vi "Find project item.vi"(8 "in (no error)":errorcluster, 9 "Item Name":string, 10 "Item Type":string, 11 "Library Refnum In":refnum<vi>) -> (0 "error out":errorcluster, 1 "Path":path, 2 "Project Item":refnum<vi>, 3 "Library Refnum Out":refnum<vi>, 5 "Found ?":bool)   [LabVIEW 2018, in "Palette Generation.lvlib"]
doc: "Find the project item reference for a particular object by name. Also returns the path to the project item."
uses:
  Palette Generation.lvlib
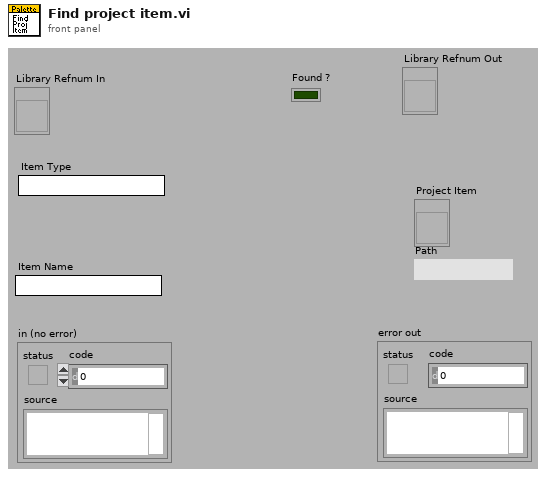
[diagram p1: front panel]
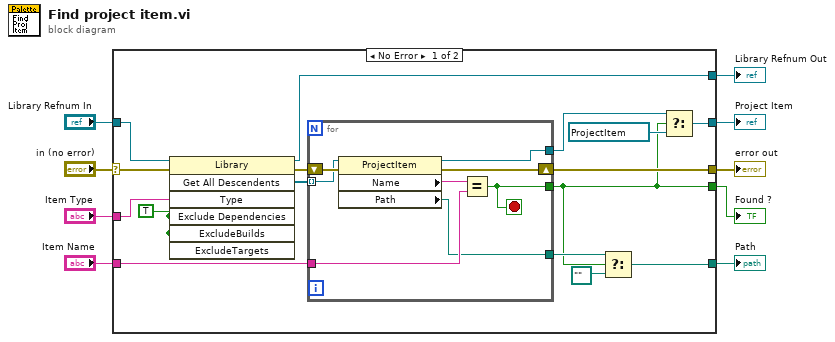
[diagram p0: block diagram]
diagram:
  n1 = case shown="No Error" "in (no error)" {
    selector: "in (no error)" -> [w10 w34]
    tunnel: [w25 w34] -> w9
    tunnel: [w24 _] -> w8
    tunnel: [w23 _] -> w7
    tunnel: "Library Refnum In" -> [w22 _]
    tunnel: "Item Name" -> [w15 _]
    tunnel: "Item Type" -> [w14 _]
    tunnel: [w12 _] -> w2
    tunnel: [w11 _] -> w1
    frame No Error {
      w13 = TRUE ("ExcludeDependencies")
      n2 = invoke class="Library" method="Get All Descendents"(reference=w22, error in=w10, "Type"=w14, "Exclude Dependencies"=w13, "ExcludeBuilds"=w13, "ExcludeTargets"=w13) -> (reference out=w12:refnum<vi>, error out=w21:errorcluster, "All Descendents"=w16:refnum<vi>[])  [unwired: 1 in, 4 out]
      n3 = for {
        tunnel: w15 -> [w29]
        shift-right: [w31] -> w25
        shift-left: w21 -> [w33]
        tunnel: w16 -> [w32] mode=indexing
        tunnel: [w28] -> w19
        tunnel: [w27] -> w17
        tunnel: [w26] -> w11
        stop <- w26 stop-if-true
        n4 = property class="ProjectItem"(reference=w32, error in=w33) -> (reference out=w27:refnum<vi>, error out=w31:errorcluster, "Name"=w30:string, "Path"=w28:path)
        n5 = Equal?(x=w30, y=w29) -> (x = y?=w26:bool)
      }
      n6 = Select(t=w19, s=w11, f=path "") -> (s? t:f=w24:path)
      n7 = Select(t=w17, s=w11, f=refnum<vi> refnum) -> (s? t:f=w23:refnum<vi>)
    }
    frame Error {
    }
  }
  "error out" <- w9
  "Path" <- w8
  "Project Item" <- w7
  "Library Refnum Out" <- w2
  "Found ?" <- w1
